vi "Actor Core.vi"(8 "error in":errorcluster, 11 "Measurement":refnum<class "Measurement.lvclass">) -> (0 "error out":errorcluster, 3 "Actor out":refnum<class "Actor.lvclass">)   [LabVIEW 2015, in "Measurement Actor.lvlib" / "Measurement.lvclass"]
doc: "This is Actor Core.vi, the main message handling loop for Actors. An actor usually just sits in this loop and processes messages as they arrive. Any error returned by the message Do.vi call will stop the loop, with error code 43 as the cannonical signal to stop with no error sent to caller. Descendants may override that in Handle Error.vi."
uses:
  Measurement.lvclass
  <vilib>/ActorFramework/Actor/Actor.lvclass
  <vilib>/ActorFramework/Actor/Actor.lvclass/Actor.ctl
  <vilib>/ActorFramework/Message Enqueuer/Message Enqueuer.lvclass/Message Enqueuer.ctl
  <vilib>/ActorFramework/Message Enqueuer/Init from Existing Queue.vi
  <vilib>/ActorFramework/Message Enqueuer/Enqueue.vi
  <vilib>/ActorFramework/Message Priority Queue/Priority Enqueue.vi
  <vilib>/ActorFramework/Message Enqueuer/Message Enqueuer.lvclass
  <vilib>/ActorFramework/Stop Msg/Stop Msg.lvclass
panel:
  out "Waveform Graph":waveform(dbl)(graph)
  out "Title":string
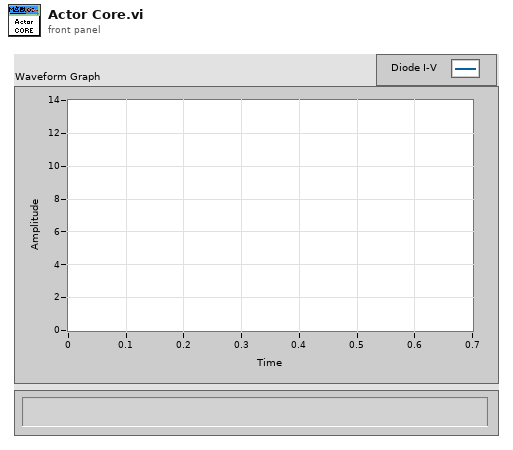
[diagram p1: front panel]
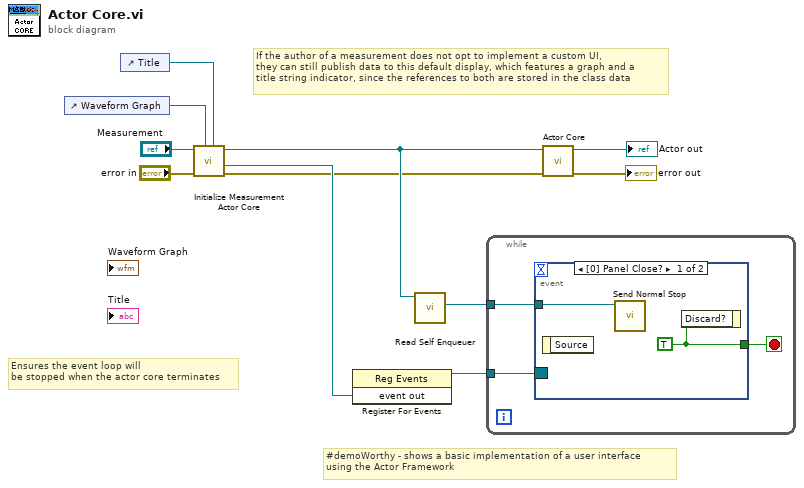
[diagram p0: block diagram]
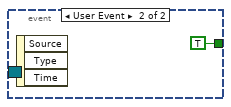
[diagram p2: hidden frame]
diagram:
  # "#demoWorthy - shows a basic implementation of a user interface\nusing the Actor Framework"
  # "Ensures the event loop will \nbe stopped when the actor core terminates"
  # "If the author of a measurement does not opt to implement a custom UI,\nthey can still publish data to this default display, which features a graph and a \ntitle string indicator, since the references to both are stored in the class data"
  n1 = control-ref of="Waveform Graph"() -> (w2:refnum<vi>)
  n2 = control-ref of="Title"() -> (w1:refnum<vi>)
  n3 = call "Initialize Measurement Actor Core.vi"("Title Ref"=w1, "Wvfm Graph Ref"=w2, "error in (no error)"="error in", "Measurement in"="Measurement") -> ("error out"=w3:errorcluster, "event out"=w6:refnum<user-event>, "Measurement out"=w4:refnum<class "Measurement.lvclass">)  [unwired: 4 in, 1 out]
  n4 = register-events(w6) -> (reference out=w5:refnum<event-registration>)  [unwired: 2 in, 1 out]
  n5 = call <vilib>:"Read Self Enqueuer.vi"("Actor"=w4) -> ("Self Enqueuer"=w7:refnum<class "Message Enqueuer.lvclass">)  [unwired: 10 in]
  n6 = while {
    tunnel: w7 -> [w14]
    tunnel: w5 -> [w12]
    stop <- w13 stop-if-true
    n7 = event shown="[0] Panel Close?" {
      selector: w12 -> [_ _]
      dyn-events: _ -> [_ _]
      timeout: _ -> [_ _]
      tunnel: w14 -> [w15 _]
      tunnel: [w16 TRUE ("Discard?")] -> w13
      event Panel Close? {
        w16 = TRUE ("Discard?")
        n8 = event-data() -> ()  [unwired: 1 in, 1 out]
        n9 = call <vilib>:"Send Normal Stop.vi"("Message Enqueuer"=w15) -> ()  [unwired: 10 in, 1 out]
        n10 = event-data("Discard?"=w16) -> ()  [unwired: 1 in, 1 out]
      }
      event User Event {
        n11 = event-data() -> ()  [unwired: 1 in, 3 out]
      }
    }
  }
  n12 = call-parent "Actor Core.vi"("error in"=w3, "Actor in"=w4) -> ("error out"=→"error out":errorcluster, "Actor out"=→"Actor out":refnum<class "Actor.lvclass">)  [unwired: 8 in]
